vi "file info extraction.vi"(0 "proceed":refnum<vi>, 11 "exp exec":T1={"data file"={"autosave"=FALSE, "File refnum"=refnum, "data file path"=path ""}, "T log file"={"File refnum"=refnum, "T log file path"=path "", "exists"=FALSE}, "exp seq"={"wave params"={"Num of avg"=0, "Num points"=1000, "Meas rate (Hz)"=100000.0}, "Setpoints"=[], "#"=-1, "index"=-1, "elapsed time (s)"=0.0, "set time (s)"=0.0, "min settle (s)"=30.0, " Exec Status"=enum."Settling"}, "error"={"status"=FALSE, "code"=0, "source"=""}}) -> (2 "message":string, 3 "T log exists":bool, 4 "T log file":path, 14 "data file exists":bool caption="data  file exists", 15 "data file":path)   [LabVIEW 2019]
doc: "This is a Bug C(T) subVI.\n\nIt extracts information about the files to display on the FP.\n\nPaul K Dixon\nP3600\nCSUSB Physics"
uses:
  typedefs/PID exec cluster.ctl
  typedefs/data file info.ctl
  typedefs/bug temp file info.ctl
  typedefs/exp seq cluster.ctl
  typedefs/wvfm acq params.ctl
  typedefs/bug meas status.ctl
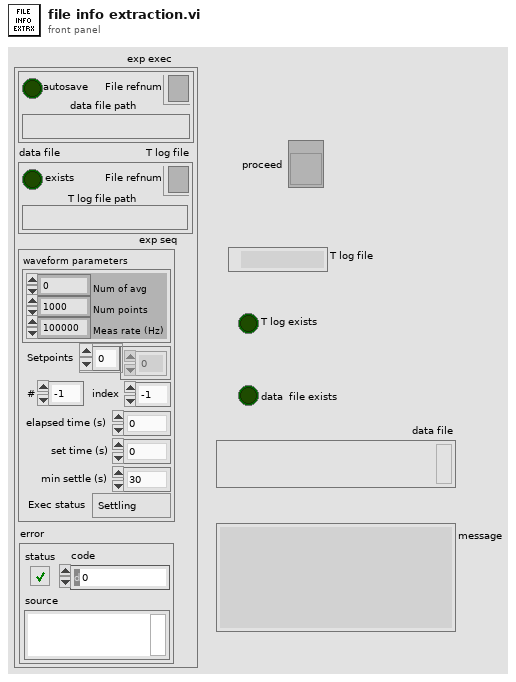
[diagram p1: front panel]
types:
  T1 = typedef "PID exec cluster.ctl" = cluster{"data file":T2, "T log file":T3, "exp seq":T4, "error":errorcluster}
  T2 = typedef "data file info.ctl" = cluster{"autosave":bool, "File refnum":refnum<file>, "data file path":path}
  T3 = typedef "bug temp file info.ctl" = cluster{"File refnum":refnum<file>, "T log file path":path, "exists":bool}
  T4 = typedef "exp seq cluster.ctl" = cluster{"wave params":T5, "Setpoints":dbl[], "#":i32, "index":i32, "elapsed time (s)":dbl, "set time (s)":dbl, "min settle (s)":dbl, " Exec Status":T6}
  T5 = typedef "wvfm acq params.ctl" = cluster{"Num of avg":i32, "Num points":i32, "Meas rate (Hz)":dbl}
  T6 = typedef "bug meas status.ctl" = enum32{"Settling", "Measuring", "Holding", "Exit"}
  T7 = enum8{"Enabled", "Disabled", "Disabled and Grayed Out"}
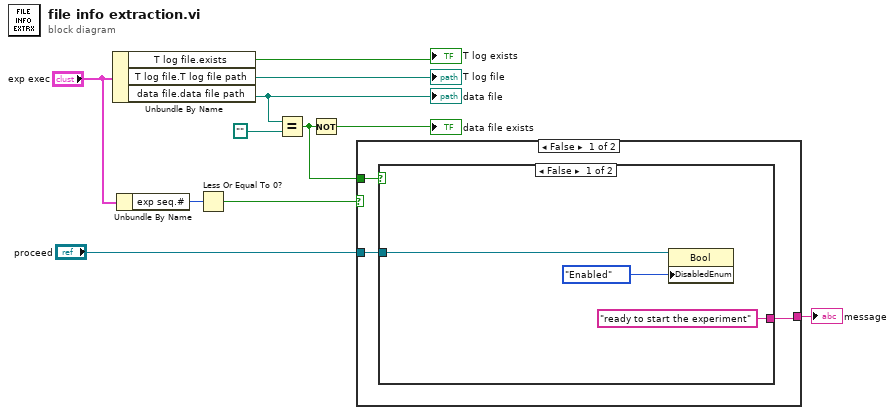
[diagram p0: block diagram]
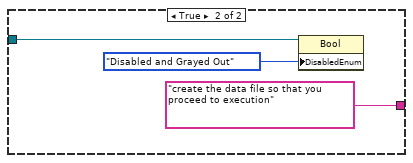
[diagram p2: hidden frame]
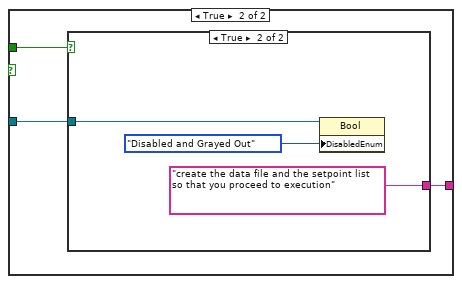
[diagram p3: hidden frame]
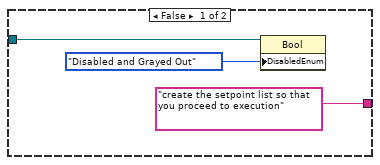
[diagram p4: hidden frame]
diagram:
  n1 = Unbundle By Name("exp exec") -> ("T log file.exists"=→"T log exists":bool, "T log file.T log file path"=→"T log file":path, "data file.data file path"=w10:path)
  "data file" <- w10
  n2 = Unbundle By Name("exp exec") -> ("exp seq.#"=w3:i32)
  n3 = Less Or Equal To 0?(x=w3) -> (x <= 0?=w2:bool)
  n4 = Equal?(x=w10, y=path "") -> (x = y?=w6:bool)
  n5 = Not(x=w6) -> (.not. x?=→"data file exists":bool)
  n6 = case shown="False" w2 {
    tunnel: "proceed" -> [w13 w23]
    tunnel: w6 -> [w12 w22]
    tunnel: [w14 w21] -> w5
    frame False {
      n7 = case shown="False" w12 {
        tunnel: ["ready to start the experiment" ("message") "create the data file so that you proceed to execution" ("message")] -> w14
        tunnel: w13 -> [w15 w18]
        frame False {
          n8 = property class="Bool"(reference=w15, "DisabledEnum"=T7."Enabled" ("Disabled")) -> ()  [unwired: 1 in, 2 out]
        }
        frame True {
          n9 = property class="Bool"(reference=w18, "DisabledEnum"=T7."Disabled and Grayed Out" ("Disabled")) -> ()  [unwired: 1 in, 2 out]
        }
      }
    }
    frame True {
      n10 = case shown="True" w22 {
        tunnel: w23 -> [w26 w29]
        tunnel: ["create the setpoint list so that you proceed to execution" ("message") "create the data file and the setpoint list so that you proceed to execution" ("message")] -> w21
        frame False {
          n11 = property class="Bool"(reference=w26, "DisabledEnum"=T7."Disabled and Grayed Out" ("Disabled")) -> ()  [unwired: 1 in, 2 out]
        }
        frame True {
          n12 = property class="Bool"(reference=w29, "DisabledEnum"=T7."Disabled and Grayed Out" ("Disabled")) -> ()  [unwired: 1 in, 2 out]
        }
      }
    }
  }
  "message" <- w5
